vi "AddToQueue.vi"(8 "error constant":errorcluster) -> (0 "error constant 2":errorcluster)   [LabVIEW 2019]
uses:
  GraphsQueue.vi
  Global.lvlib
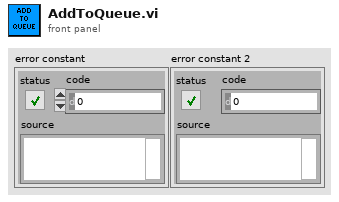
[diagram p1: front panel]
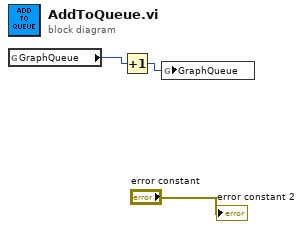
[diagram p0: block diagram]
diagram:
  n1 = global read "GraphsQueue.vi" "GraphQueue"() -> (w3:i16)
  n2 = Increment(x=w3) -> (x+1=w2:i16)
  n3 = global write "GraphsQueue.vi" "GraphQueue"(w2) -> ()
  "error constant 2" <- "error constant"
